vi "2_AdvancedDemo_MHHisto.vi"() -> ()   [LabVIEW 2017]
uses:
  Types/MH_InputChannel.ctl
  Types/MH_UIThread_Cmds.ctl
  Types/MH_UIThread_Data.ctl
  _lib/PQ/MultiHarp/MH_InitInfo.ctl
  Types/MH_SetInpChanData.ctl
  Types/MH_SetInpChanCmds.ctl
  _lib/PQ/MultiHarp/MH_RefSource.ctl
  _lib/PQ/MultiHarp/MH_MeasMode.ctl
  <vilib>/Utility/error.llb/DialogType.ctl
  <vilib>/Utility/error.llb/Error Cluster From Error Code.vi
  _lib/PQ/MultiHarp/MH_LibVersion_global.vi
  _lib/PQ/MultiHarp/mhlib_x86_x64_UIThread.llb/MH_DllPath_global.vi
  <vilib>/ErrorRing/Error Ring.xnode
panel:
  in  "Settings":bool=TRUE
  in  "Run continuously":bool=TRUE caption="Conti."
  in  "Start":bool
  in  "Scale":bool
  out "CountRates":i32[](graph)
  in  "AllChannels":T1={"Enable"=TRUE, "Offset"=0, "Level"=-100, "Edge"=0, "DeadTime"=1000, "UseDeadTime"=FALSE, "SetEnableAllChan"=TRUE, "SetEdgeAllChan"=TRUE, "SetLevelAllChan"=TRUE, "SetOffsetAllChan"=TRUE, "SetUseDTAllChan"=TRUE, "SetDeadTAllChan"=TRUE} {"DeadTime" min=800 max=160000 step=1; "Edge" items=["falling", "rising"]; "Offset" min=-100000 max=100000 step=10; "Level" min=-1200 max=1200 step=1}
  in  "HistoLength":i32(ring)=6 caption="Num Bins" items=["1024", "2048", "4096", "8192", "16384", "32768", "65536"]
  in  "OvlLevel":u32=4294967295 caption="Ovl.Level" min=1 step=1
  in  "StopOvl.":bool=TRUE
  in  "AcqTime":i32=1000 caption="Acqu.           ms" min=1 max=360000 step=1
  in  "Binning":i32(ring) caption="Resol.            ps" items=["10", "20", "40", "80", "160", "320", "640", "1280", "2560", "5120", "10240", "20480", "40960", "81920", "163840", "327680", "655360", "1310720", "2621440", "5242880", "10485760", "20971520", "41943040"]
  in  "HistoOffset":i32 caption="Offset            ns" min=0 max=100000000 step=1
  out "HistoGraph":T2(graph)={0.0, "Resolution"=0.08, "Histogram"=[]}
  in  "SyncDeadTime":i32=1000 caption="Dead T.   ps" min=800 max=160000 step=1
  in  "UseDeadTime":bool caption="Use DT."
  in  "SyncEdge":i32(ring) caption="Edge" items=["falling", "rising"]
  in  "SyncDivider":i32(ring) caption="Divider" items=["1", "2", "4", "8", "16"]
  in  "SyncOffset":i32 caption="Offset      ps" min=-100000 max=100000 step=10
  in  "SyncLevel":i32=-100 caption="Level      mV" min=-1200 max=1200 step=1
  in  "Channels":T3[](array[typedef])=[{"Name"="Inp.Chan 1", "Enable"=TRUE, "Edge"=0, "Level"=-100, "Offset"=0, "UseDeadTime"=FALSE, "DeadTime"=1000}, {"Name"="Inp.Chan 2", "Enable"=TRUE, "Edge"=0, "Level"=-100, "Offset"=0, "UseDeadTime"=FALSE, "DeadTime"=1000}, {"Name"="Inp.Chan 3", "Enable"=TRUE, "Edge"=0, "Level"=-100, "Offset"=0, "UseDeadTime"=FALSE, "DeadTime"=1000}, {"Name"="Inp.Chan 4", "Enable"=TRUE, "Edge"=0, "Level"=-100, "Offset"=0, "UseDeadTime"=FALSE, "DeadTime"=1000}, {"Name"="Inp.Chan 5", "Enable"=TRUE, "Edge"=0, "Level"=-100, "Offset"=0, "UseDeadTime"=FALSE, "DeadTime"=1000}, {"Name"="Inp.Chan 6", "Enable"=TRUE, "Edge"=0, "Level"=-100, "Offset"=0, "UseDeadTime"=FALSE, "DeadTime"=1000}, {"Name"="Inp.Chan 7", "Enable"=TRUE, "Edge"=0, "Level"=-100, "Offset"=0, "UseDeadTime"=FALSE, "DeadTime"=1000}, {"Name"="Inp.Chan 8", "Enable"=TRUE, "Edge"=0, "Level"=-100, "Offset"=0, "UseDeadTime"=FALSE, "DeadTime"=1000}, {"Name"="Inp.Chan 9", "Enable"=TRUE, "Edge"=0, "Level"=-100, "Offset"=0, "UseDeadTime"=FALSE, "DeadTime"=1000}, {"Name"="Inp.Chan 10", "Enable"=TRUE, "Edge"=0, "Level"=-100, "Offset"=0, "UseDeadTime"=FALSE, "DeadTime"=1000}, {"Name"="Inp.Chan 11", "Enable"=TRUE, "Edge"=0, "Level"=-100, "Offset"=0, "UseDeadTime"=FALSE, "DeadTime"=1000}, {"Name"="Inp.Chan 12", "Enable"=TRUE, "Edge"=0, "Level"=-100, "Offset"=0, "UseDeadTime"=FALSE, "DeadTime"=1000}, {"Name"="Inp.Chan 13", "Enable"=TRUE, "Edge"=0, "Level"=-100, "Offset"=0, "UseDeadTime"=FALSE, "DeadTime"=1000}, {"Name"="Inp.Chan 14", "Enable"=TRUE, "Edge"=0, "Level"=-100, "Offset"=0, "UseDeadTime"=FALSE, "DeadTime"=1000}, {"Name"="Inp.Chan 15", "Enable"=TRUE, "Edge"=0, "Level"=-100, "Offset"=0, "UseDeadTime"=FALSE, "DeadTime"=1000}, {"Name"="Inp.Chan 16", "Enable"=TRUE, "Edge"=0, "Level"=-100, "Offset"=0, "UseDeadTime"=FALSE, "DeadTime"=1000}] {"DeadTime" min=800 max=160000 step=1; "Edge" items=["falling", "rising"]; "Offset" min=-100000 max=100000 step=10; "Level" min=-1200 max=1200 step=1}
  out "SyncRate":string="Sync Rate: 4999950 cps\n"
  out "OverFlow":bool caption="Overflow:"
  out "Status":string="Readout Rate: 8.6 Hz\t\tTotal Counts:\t\tCh. 1: 0 cnts.\t\tCh. 2: 1962112 cnts.\t\tCh. 3: 0 cnts.\t\tCh. 4: 1962112 cnts.\t\tCh. 5: 0 cnts.\t\tCh. 6: 1962112 cnts.\t\tCh. 7: 0 cnts.\t\tCh. 8: 1962112 cnts.\t\tCh. 9: 1962113 cnts.\t\tCh.10: 0 cnts.\t\tCh.11: 1962113 cnts.\t\tCh.12: 0 cnts.\t\tCh.13: 1962113 cnts.\t\tCh.14: 0 cnts.\t\tCh.15: 1962113 cnts.\t\tCh.16: 1962113 cnts.\t\t"
  # "Acquisition"
  # "All Channels"
  # "Sync"
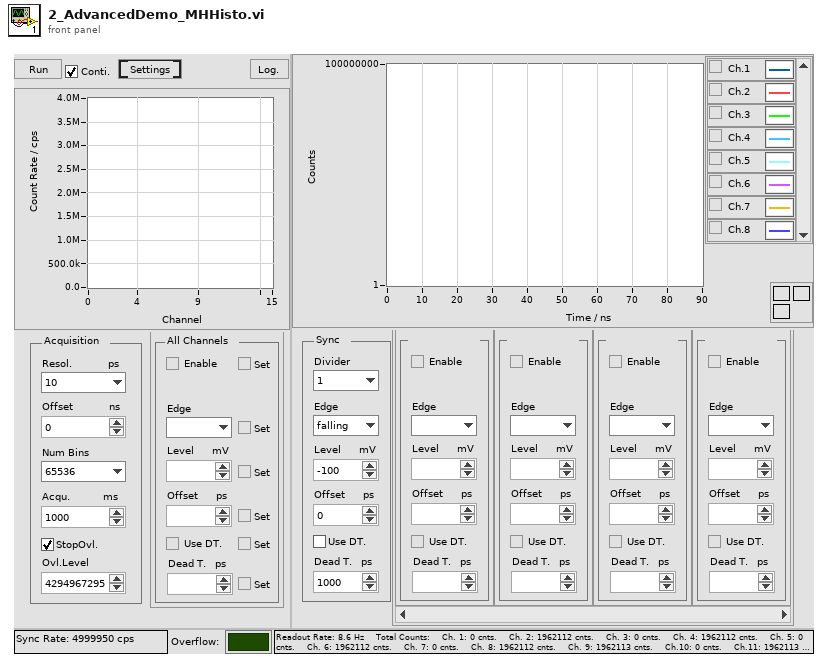
[diagram p1: front panel]
types:
  T1 = cluster{"Enable":bool, "Offset":i32, "Level":i32, "Edge":i32, "DeadTime":i32, "UseDeadTime":bool, "SetEnableAllChan":bool, "SetEdgeAllChan":bool, "SetLevelAllChan":bool, "SetOffsetAllChan":bool, "SetUseDTAllChan":bool, "SetDeadTAllChan":bool}
  T2 = cluster{dbl, "Resolution":dbl, "Histogram":u32[][]}
  T3 = typedef "MH_InputChannel.ctl" = cluster{"Name":string, "Enable":bool, "Edge":i32, "Level":i32, "Offset":i32, "UseDeadTime":bool, "DeadTime":i32}
  T4 = typedef "MH_UIThread_Data.ctl" = cluster{"Init Info":T5, "DevIdx":i32, "SyncDivider":i32, "SyncOffset":i32, "SyncLevel":i32, "Channels":T3[], "CurrentChannels":i32[], "AcqTime":i32, "Binning":i32, "HistoOffset":i32, "HistoLen":i32, "StopOvl.":bool, "OvlLevel":u32, "SyncEdge":i32, "StartMeas":bool, "HistoLength":i32, "Resolution":dbl, "Run cont.":bool, "Status":string, "SyncRate":i32, "BitShift":i32, "HistoAcqTime":dbl, "SyncRateStart":i32, "UseDeadTime":bool, "SyncDeadTime":i32, "SetInpChan":T6[]}
  T5 = typedef "MH_InitInfo.ctl" = cluster{"Library Version":string, "Serial No.":string, "Model":string, "Partnum":string, "Version":string, "features":i32, "nchannels":i32, "Base Resolution":dbl, "Bin Steps":i32}
  T6 = typedef "MH_SetInpChanData.ctl" = cluster{"Channel":i32, "Cmds":T7[], "Changed":cluster{"Name":bool, "Enable":bool, "Edge":bool, "Level":bool, "Offset":bool, "UseDeadTime":bool, "DeadTime":bool}}
  T7 = typedef "MH_SetInpChanCmds.ctl" = enum16{"SetInpChanEnable", "SetInpChanOffset", "SetInpChanDeadTime", "SetInpChanTrg"}
  T8 = typedef "MH_UIThread_Cmds.ctl" = enum16{"Idle", "Init", "SetInpChan", "SetSyncDivider", "SetSyncTrg", "SetSyncOffset", "SetSyncDeadTime", "SetBinning", "SetHistoOffset", "SetHistoLen", "SetStopOvl", "SetBitShift", "SetHistoAcqTime", "GetRates", "GetAllRates", "StartMeas", "StopMeas", "AbortMeas", "GetResolution", "GetHistos", "GetAllHistos", "ReadFiFo", "WriteStatus", "Resize", "EnableControls", "DisableControls", "Error", "Exit"}
  T9 = enum8{"Enabled", "Disabled", "Disabled and Grayed Out"}
  T10 = cluster{"[0]":bool, "[1]":bool, "[2]":bool, "[3]":bool, "[4]":bool, "[5]":bool}
  T11 = typedef "MH_MeasMode.ctl" = i32
  T12 = typedef "MH_RefSource.ctl" = enum16{"INTERNAL", "EXTERNAL_10MHZ", "WR_MASTER_GENERIC", "WR_SLAVE_GENERIC", "WR_GRANDM_GENERIC", "EXTN_GPS_PPS", "EXTN_GPS_PPS_UART", "WR_MASTER_MHARP", "WR_SLAVE_MHARP", "WR_GRANDM_MHARP"}
  T13 = cluster{dbl, "Resolution":dbl, "Histograms":u32[][]}
  T14 = typedef "DialogType.ctl" = u16
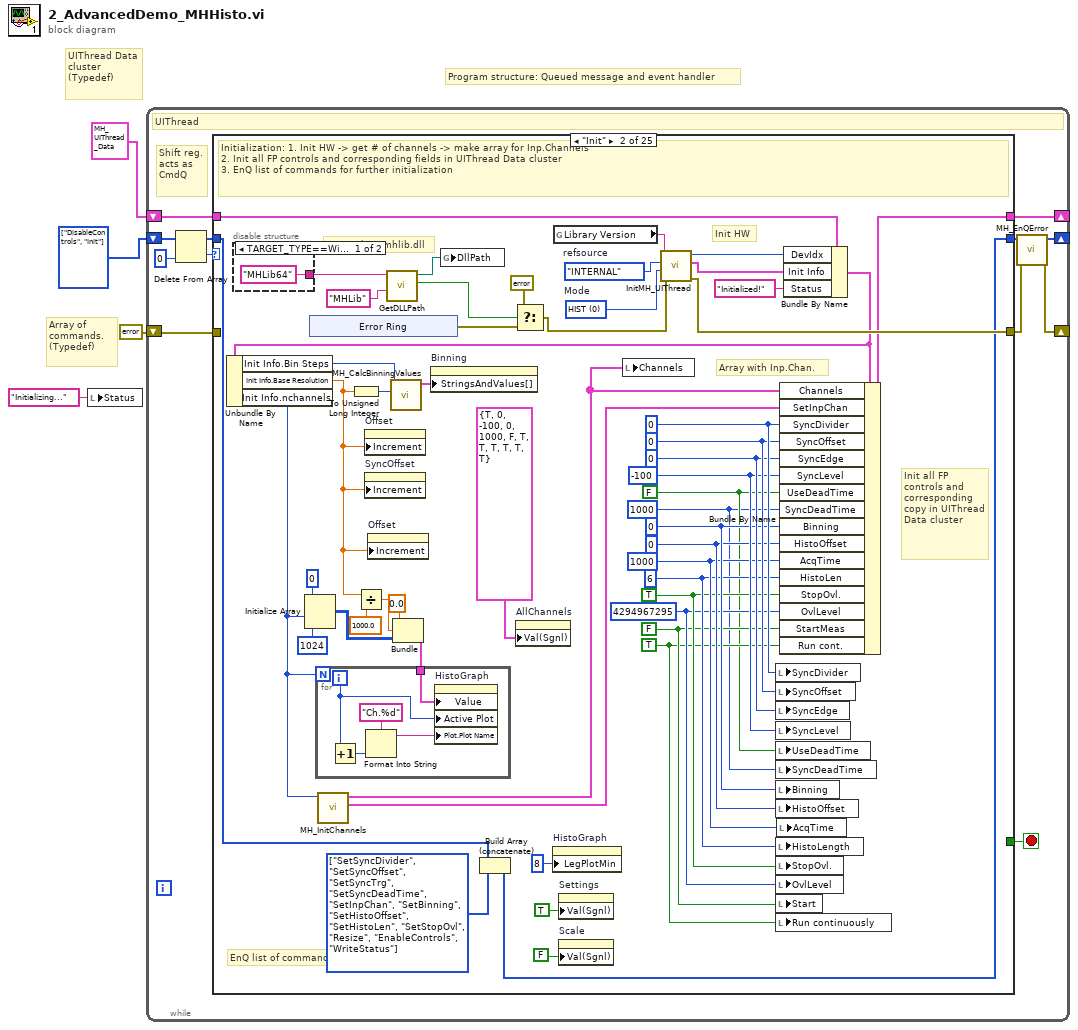
[diagram p0: block diagram]
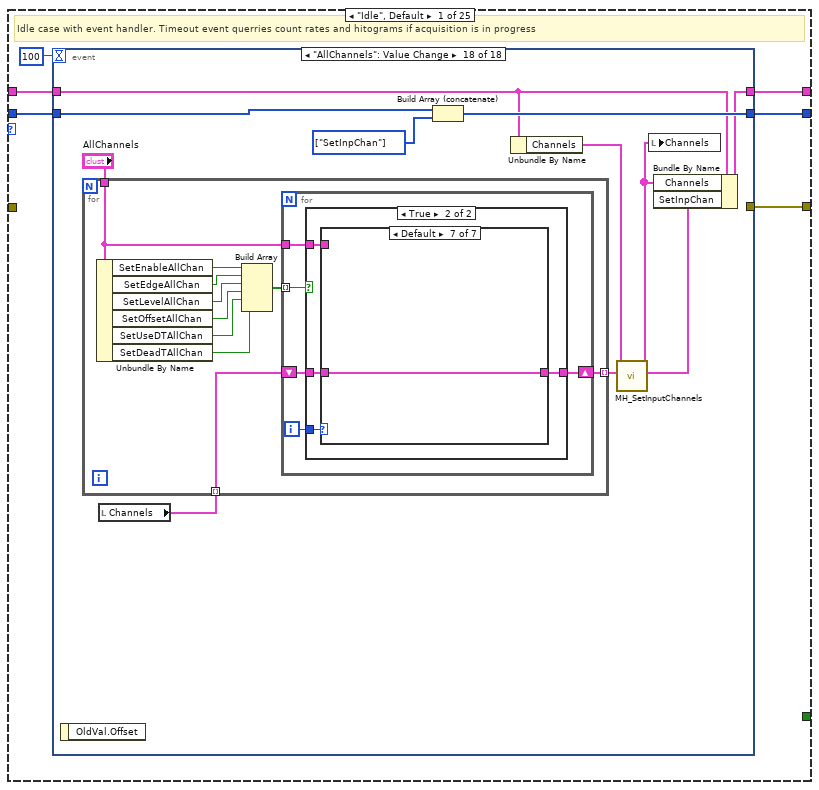
[diagram p2: hidden frame]
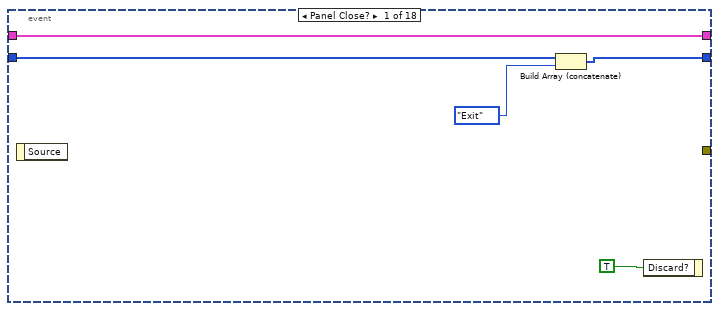
[diagram p3: hidden frame]
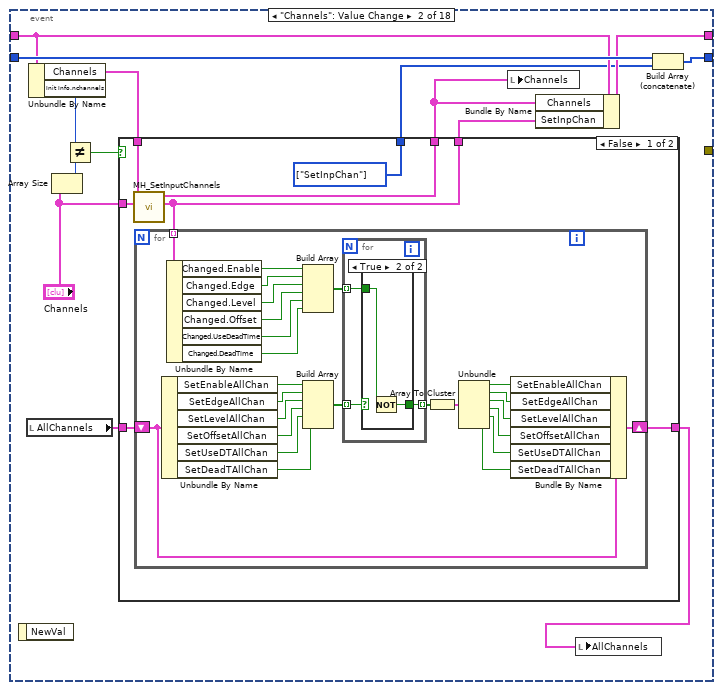
[diagram p4: hidden frame]
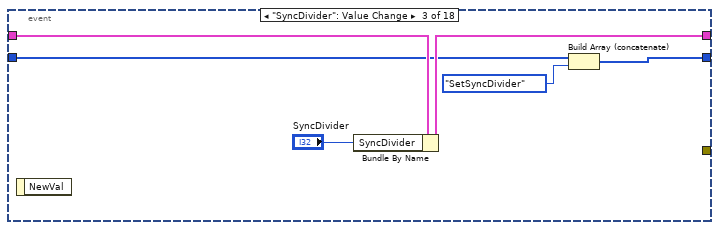
[diagram p7: hidden frame]
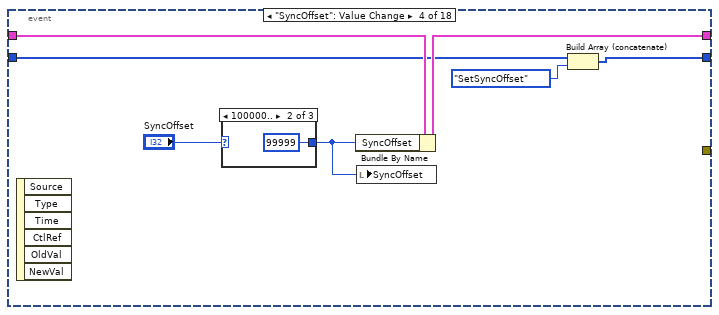
[diagram p8: hidden frame]
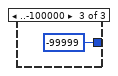
[diagram p10: hidden frame]
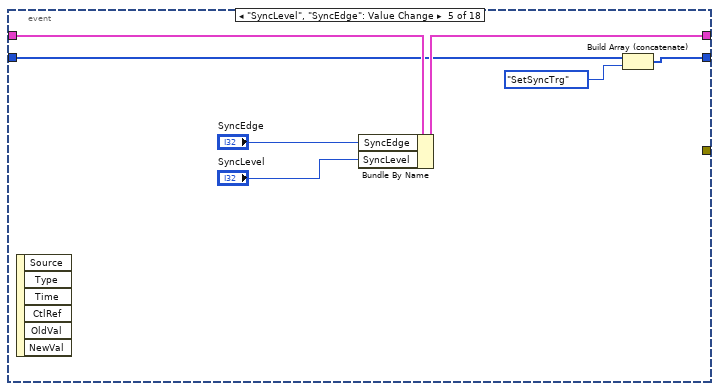
[diagram p11: hidden frame]
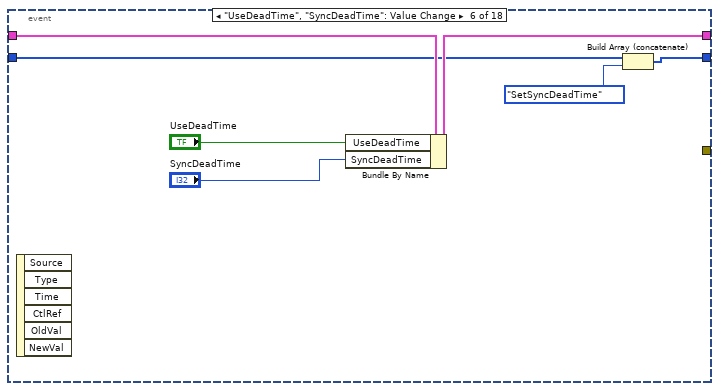
[diagram p12: hidden frame]
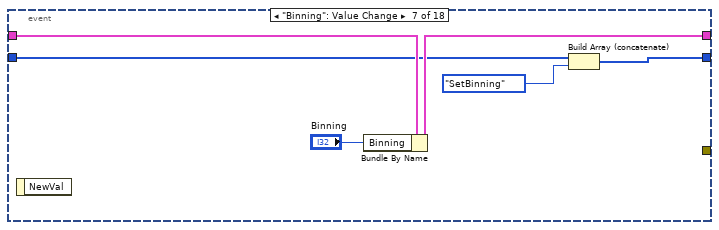
[diagram p13: hidden frame]
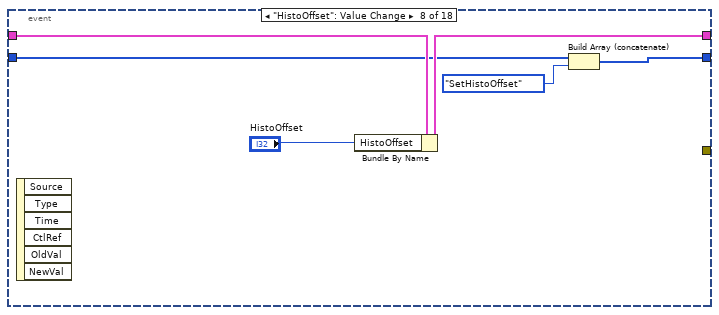
[diagram p14: hidden frame]
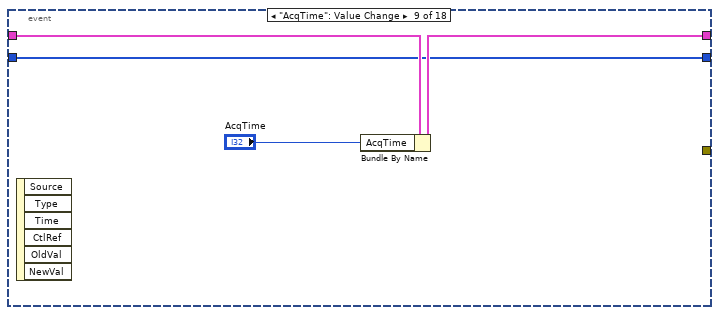
[diagram p15: hidden frame]
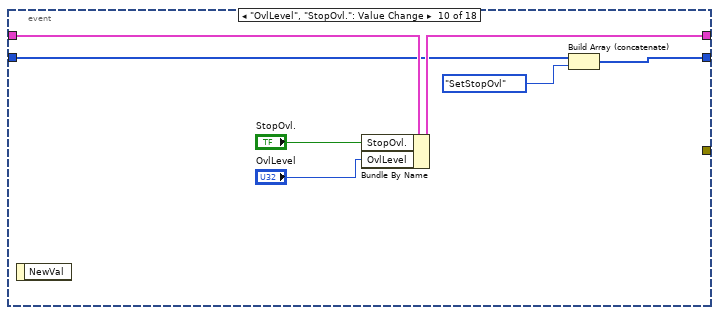
[diagram p16: hidden frame]
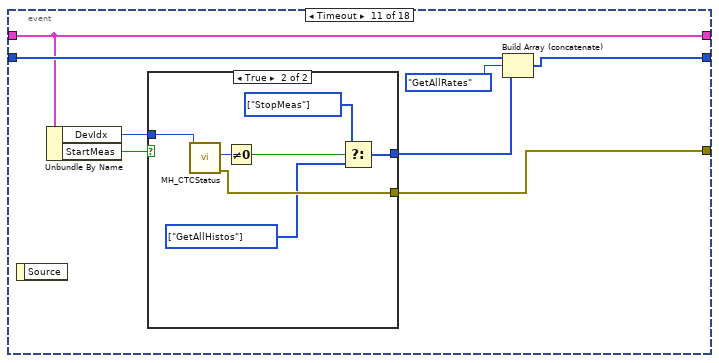
[diagram p17: hidden frame]
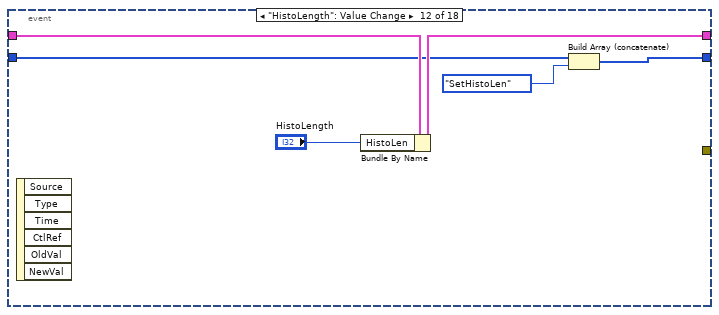
[diagram p19: hidden frame]
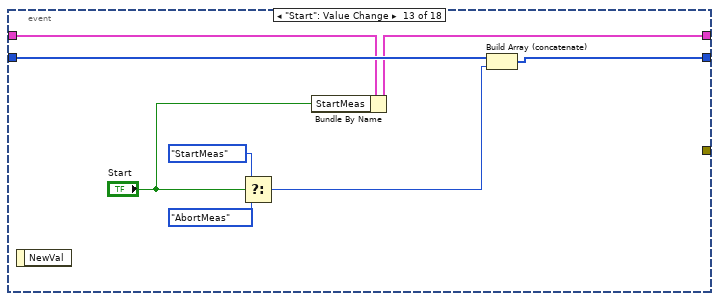
[diagram p20: hidden frame]
diagram:
  w3 = T8[] [enum."DisableControls", enum."Init"] items=["Idle", "Init", "SetInpChan", "SetSyncDivider", "SetSyncTrg", "SetSyncOffset", "SetSyncDeadTime", "SetBinning", "SetHistoOffset", "SetHistoLen", "SetStopOvl", "SetBitShift", "SetHistoAcqTime", "GetRates", "GetAllRates", "StartMeas", "StopMeas", "AbortMeas", "GetResolution", "GetHistos", "GetAllHistos", "ReadFiFo", "WriteStatus", "Resize", "EnableControls", "DisableControls", "Error", "Exit"]
  # "Array of commands.\n(Typedef)"
  # "Program structure: Queued message and event handler"
  # "UIThread Data cluster\n(Typedef)"
  n1 = local write "Status"("Initializing..." ("Status")) -> ()
  n2 = while {
    shift-right: [w5] -> _
    shift-left: w3 -> [w12]
    shift-right: [w15] -> _
    shift-left: T4 {"Init Info"={"Library Version"="", "Serial No."="", "Model"="", "Partnum"="", "Version"="", "features"=0, "nchannels"=0, "Base Resolution"=0.0, "Bin Steps"=0}, "DevIdx"=0, "SyncDivider"=1, "SyncOffset"=0, "SyncLevel"=50, "Channels"=[], "CurrentChannels"=[], "AcqTime"=1, "Binning"=1, "HistoOffset"=1, "HistoLen"=1024, "StopOvl."=FALSE, "OvlLevel"=1024, "SyncEdge"=10, "StartMeas"=FALSE, "HistoLength"=0, "Resolution"=0.0, "Run cont."=FALSE, "Status"="", "SyncRate"=0, "BitShift"=0, "HistoAcqTime"=0.0, "SyncRateStart"=0, "UseDeadTime"=FALSE, "SyncDeadTime"=800, "SetInpChan"=[]} -> [w14]
    shift-right: [w7] -> _
    shift-left: errorcluster {"status"=FALSE, "code"=0, "source"=""} ("error IO") -> [w13]
    stop <- w16 stop-if-true
    # "Shift reg.\nacts as\nCmdQ"
    # "UIThread"
    n3 = Delete From Array(array=w12, index=0) -> (deleted portion=w10:T8, array with subset deleted=w9:T8[])  [unwired: 1 in]
    n4 = case shown="\"Init\"" w10 {
      tunnel: [w22 w301 w325 w387 w396 w408 w414 w421 w429 w437 w442 w453 w464 w479 w487 w501 w515 w540 w572 w596 w609 w616 w628 w634 w638] -> w6
      tunnel: [_ _ _ _ _ _ _ _ _ _ _ _ _ _ _ _ _ _ _ _ _ _ _ _ TRUE] -> w16
      tunnel: [w21 w281 w326 w389 w397 w409 w418 w425 w430 w432 w443 w452 w463 w485 w490 w504 w511 w539 w571 w595 w597 w615 w627 w635 w641] -> w15
      tunnel: w14 -> [w20 w286 w326 w389 w397 w409 w418 w425 w430 w433 w443 w452 w463 w485 w491 w505 w512 w539 w571 w595 w597 w615 w627 w635 w641]
      tunnel: [w17 w304 w323 w385 w395 w407 w417 w424 w428 w436 w441 w446 w462 w484 w493 w507 w513 w537 w567 _ _ _ _ _ w639] -> w8
      tunnel: w13 -> [_ _ _ _ _ _ _ _ _ _ _ _ _ _ _ _ _ _ _ _ _ _ _ w636 _]
      tunnel: w9 -> [w19 w303 w325 w387 w396 w408 w414 w420 w429 w437 w442 w453 w464 w480 w488 w502 w515 w540 w572 w596 w609 w616 w628 _ w638]
      frame "Idle", Default {
        # "Idle case with event handler. Timeout event querries count rates and hitograms if acquisition is in progress"
        n5 = event shown="[17] \"AllChannels\": Value Change" {
          selector: _ -> [_ _ _ _ _ _ _ _ _ _ _ _ _ _ _ _ _ _]
          dyn-events: _ -> [_ _ _ _ _ _ _ _ _ _ _ _ _ _ _ _ _ _]
          timeout: 100 -> [_ _ _ _ _ _ _ _ _ _ _ _ _ _ _ _ _ _]
          tunnel: [w23 w40 w82 w90 w99 w107 w113 w119 w124 w130 w140 w151 w159 w167 w173 w181 w191 w204] -> w22
          tunnel: [w26 w33 w86 w93 w103 w110 w116 w122 w126 w133 w139 w154 w157 w165 w172 w180 w194 w198] -> w21
          tunnel: w20 -> [w26 w35 w87 w94 w104 w111 w117 w123 w127 w134 w139 w155 w158 w166 w172 w180 w194 w199]
          tunnel: w19 -> [w25 w41 w84 w92 w101 w109 w115 w121 w124 w132 w142 w153 w161 w167 w173 w181 w192 w205]
          tunnel: [_ _ _ _ _ _ _ _ _ _ w135 _ _ _ _ _ _ _] -> w17
          event Panel Close? {
            n6 = event-data() -> ()  [unwired: 1 in, 1 out]
            n7 = Build Array (concatenate)(w25, MH_UIThread_Cmds."Exit") -> (w23:T8[])
            n8 = event-data("Discard?"=TRUE) -> ()  [unwired: 1 in, 1 out]
          }
          event "Channels": Value Change {
            n9 = event-data() -> ()  [unwired: 1 in, 1 out]
            n10 = local read "AllChannels"() -> (w29:T1)
            n11 = Unbundle By Name(w35) -> ("Channels"=w36:T3[], "Init Info.nchannels"=w39:i32)
            n12 = Array Size(array="Channels") -> (size(s)=w38:i32)
            n13 = Not Equal?(x=w39, y=w38) -> (x != y?=w37:bool)
            n14 = case shown="False" w37 {
              tunnel: "Channels" -> [w47 _]
              tunnel: [w46 w81] -> w34
              tunnel: w36 -> [w48 w81]
              tunnel: [w44 _] -> w32
              tunnel: [w45 _] -> w30
              tunnel: w29 -> [w43 w80]
              tunnel: [w42 w80] -> w28
              frame False {
                w45 = T8[] [enum."SetInpChan"] items=["Idle", "Init", "SetInpChan", "SetSyncDivider", "SetSyncTrg", "SetSyncOffset", "SetSyncDeadTime", "SetBinning", "SetHistoOffset", "SetHistoLen", "SetStopOvl", "SetBitShift", "SetHistoAcqTime", "GetRates", "GetAllRates", "StartMeas", "StopMeas", "AbortMeas", "GetResolution", "GetHistos", "GetAllHistos", "ReadFiFo", "WriteStatus", "Resize", "EnableControls", "DisableControls", "Error", "Exit"] ("array")
                n15 = call "MH_SetInputChannels.vi"("Channels new"=w47, "Channels old"=w48) -> ("SetInpChan"=w44:T6[], "Channels"=w46:T3[])  [unwired: 8 in]
                n16 = for {
                  tunnel: w44 -> [w73] mode=indexing
                  shift-right: [w55] -> w42
                  shift-left: w43 -> [w57]
                  n17 = Unbundle By Name(w57) -> ("SetEnableAllChan"=w66:bool, "SetEdgeAllChan"=w65:bool, "SetLevelAllChan"=w64:bool, "SetOffsetAllChan"=w63:bool, "SetUseDTAllChan"=w62:bool, "SetDeadTAllChan"=w61:bool)
                  n18 = Unbundle By Name(w73) -> ("Changed.Enable"=w72:bool, "Changed.Edge"=w71:bool, "Changed.Level"=w70:bool, "Changed.Offset"=w69:bool, "Changed.UseDeadTime"=w68:bool, "Changed.DeadTime"=w67:bool)
                  n19 = Build Array(w72, w71, w70, w69, w68, w67) -> (w59:bool[])
                  n20 = Build Array(w66, w65, w64, w63, w62, w61) -> (w60:bool[])
                  n21 = for {
                    tunnel: w60 -> [w76] mode=indexing
                    tunnel: w59 -> [w74] mode=indexing
                    tunnel: [w75] -> w58 mode=indexing
                    n22 = case shown="True" w76 {
                      selector: w76 -> [w77 _]
                      tunnel: [w77 w78] -> w75
                      tunnel: w74 -> [_ w79]
                      frame False {
                      }
                      frame True {
                        n23 = Not(x=w79) -> (.not. x?=w78:bool)
                      }
                    }
                  }
                  n24 = Array To Cluster(array=w58) -> (cluster=w56:T10)
                  n25 = Unbundle(w56) -> ("[0]"=w54:bool, "[1]"=w53:bool, "[2]"=w52:bool, "[3]"=w51:bool, "[4]"=w50:bool, "[5]"=w49:bool)
                  n26 = Bundle By Name(cluster=w57, "SetEnableAllChan"=w54, "SetEdgeAllChan"=w53, "SetLevelAllChan"=w52, "SetOffsetAllChan"=w51, "SetUseDTAllChan"=w50, "SetDeadTAllChan"=w49) -> (w55:T1)
                }
              }
              frame True {
              }
            }
            n27 = local write "Channels"(w34) -> ()
            n28 = Bundle By Name(cluster=w35, "Channels"=w34, "SetInpChan"=w32) -> (w33:T4)
            n29 = local write "AllChannels"(w28) -> ()
            n30 = Build Array (concatenate)(w41, w30) -> (w40:T8[])
          }
          event "SyncDivider": Value Change {
            n31 = event-data() -> ()  [unwired: 1 in, 1 out]
            n32 = Bundle By Name(cluster=w87, "SyncDivider"="SyncDivider") -> (w86:T4)
            n33 = Build Array (concatenate)(w84, MH_UIThread_Cmds."SetSyncDivider") -> (w82:T8[])
          }
          event "SyncOffset": Value Change {
            n34 = event-data() -> ()  [unwired: 1 in, 6 out]
            n35 = case shown="100000.." "SyncOffset" {
              selector: "SyncOffset" -> [w95 _ _]
              tunnel: [w95 99999 ("SyncOffset") -99999 ("SyncOffset")] -> w88
              frame Default {
              }
              frame 100000.. {
              }
              frame ..-100000 {
              }
            }
            n36 = Bundle By Name(cluster=w94, "SyncOffset"=w88) -> (w93:T4)
            n37 = local write "SyncOffset"(w88) -> ()
            n38 = Build Array (concatenate)(w92, MH_UIThread_Cmds."SetSyncOffset") -> (w90:T8[])
          }
          event "SyncLevel", "SyncEdge": Value Change {
            n39 = event-data() -> ()  [unwired: 1 in, 6 out]
            n40 = Bundle By Name(cluster=w104, "SyncEdge"="SyncEdge", "SyncLevel"="SyncLevel") -> (w103:T4)
            n41 = Build Array (concatenate)(w101, MH_UIThread_Cmds."SetSyncTrg") -> (w99:T8[])
          }
          event "UseDeadTime", "SyncDeadTime": Value Change {
            n42 = event-data() -> ()  [unwired: 1 in, 6 out]
            n43 = Bundle By Name(cluster=w111, "UseDeadTime"="UseDeadTime", "SyncDeadTime"="SyncDeadTime") -> (w110:T4)
            n44 = Build Array (concatenate)(w109, MH_UIThread_Cmds."SetSyncDeadTime") -> (w107:T8[])
          }
          event "Binning": Value Change {
            n45 = event-data() -> ()  [unwired: 1 in, 1 out]
            n46 = Bundle By Name(cluster=w117, "Binning"="Binning") -> (w116:T4)
            n47 = Build Array (concatenate)(w115, MH_UIThread_Cmds."SetBinning") -> (w113:T8[])
          }
          event "HistoOffset": Value Change {
            n48 = event-data() -> ()  [unwired: 1 in, 6 out]
            n49 = Bundle By Name(cluster=w123, "HistoOffset"="HistoOffset") -> (w122:T4)
            n50 = Build Array (concatenate)(w121, MH_UIThread_Cmds."SetHistoOffset") -> (w119:T8[])
          }
          event "AcqTime": Value Change {
            n51 = event-data() -> ()  [unwired: 1 in, 6 out]
            n52 = Bundle By Name(cluster=w127, "AcqTime"="AcqTime") -> (w126:T4)
          }
          event "OvlLevel", "StopOvl.": Value Change {
            n53 = event-data() -> ()  [unwired: 1 in, 1 out]
            n54 = Bundle By Name(cluster=w134, "StopOvl."="StopOvl.", "OvlLevel"="OvlLevel") -> (w133:T4)
            n55 = Build Array (concatenate)(w132, MH_UIThread_Cmds."SetStopOvl") -> (w130:T8[])
          }
          event Timeout {
            n56 = event-data() -> ()  [unwired: 1 in, 1 out]
            n57 = Unbundle By Name(w139) -> ("DevIdx"=w137:i32, "StartMeas"=w138:bool)
            n58 = case shown="True" w138 {
              tunnel: w137 -> [_ w149]
              tunnel: [_ w147] -> w136
              tunnel: [_ w145] -> w135
              frame False {
              }
              frame True {
                w143 = T8[] [enum."GetAllHistos"] items=["Idle", "Init", "SetInpChan", "SetSyncDivider", "SetSyncTrg", "SetSyncOffset", "SetSyncDeadTime", "SetBinning", "SetHistoOffset", "SetHistoLen", "SetStopOvl", "SetBitShift", "SetHistoAcqTime", "GetRates", "GetAllRates", "StartMeas", "StopMeas", "AbortMeas", "GetResolution", "GetHistos", "GetAllHistos", "ReadFiFo", "WriteStatus", "Resize", "EnableControls", "DisableControls", "Error", "Exit"]
                w146 = T8[] [enum."StopMeas"] items=["Idle", "Init", "SetInpChan", "SetSyncDivider", "SetSyncTrg", "SetSyncOffset", "SetSyncDeadTime", "SetBinning", "SetHistoOffset", "SetHistoLen", "SetStopOvl", "SetBitShift", "SetHistoAcqTime", "GetRates", "GetAllRates", "StartMeas", "StopMeas", "AbortMeas", "GetResolution", "GetHistos", "GetAllHistos", "ReadFiFo", "WriteStatus", "Resize", "EnableControls", "DisableControls", "Error", "Exit"]
                n59 = call "MH_CTCStatus.vi"("devidx"=w149) -> ("error out"=w145:errorcluster, "ctcstatus"=w148:i32)  [unwired: 8 in, 1 out]
                n60 = Not Equal To 0?(x=w148) -> (x != 0?=w144:bool)
                n61 = Select(t=w146, s=w144, f=w143) -> (s? t:f=w147:T8[])
              }
            }
            n62 = Build Array (concatenate)(w142, MH_UIThread_Cmds."GetAllRates", w136) -> (w140:T8[])
          }
          event "HistoLength": Value Change {
            n63 = event-data() -> ()  [unwired: 1 in, 6 out]
            n64 = Bundle By Name(cluster=w155, "HistoLen"="HistoLength") -> (w154:T4)
            n65 = Build Array (concatenate)(w153, MH_UIThread_Cmds."SetHistoLen") -> (w151:T8[])
          }
          event "Start": Value Change {
            n66 = event-data() -> ()  [unwired: 1 in, 1 out]
            n67 = Select(t=MH_UIThread_Cmds."StartMeas", s="Start", f=MH_UIThread_Cmds."AbortMeas") -> (s? t:f=w160:T8)
            n68 = Bundle By Name(cluster=w158, "StartMeas"="Start") -> (w157:T4)
            n69 = Build Array (concatenate)(w161, w160) -> (w159:T8[])
          }
          event "Run continuously": Value Change {
            n70 = event-data() -> ()  [unwired: 1 in, 1 out]
            n71 = Bundle By Name(cluster=w166, "Run cont."="Run continuously") -> (w165:T4)
          }
          event "Scale": Value Change {
            n72 = event-data() -> ()  [unwired: 1 in, 1 out]
            n73 = Select(t=u8 0 ("Y Scale.Mapping Mode"), s="Scale", f=u8 1 ("Y Scale.Mapping Mode")) -> (s? t:f=w168:u8)
            n74 = property on="HistoGraph" class="WFGraph (strict)"("YScale.Mapping Mode"=w168) -> ()  [unwired: 2 in, 2 out]
          }
          event "Settings": Value Change {
            n75 = event-data() -> ()  [unwired: 1 in, 1 out]
            n76 = property on="Splitter" class="Splitter"() -> ("Position"=w179:i32)  [unwired: 2 in, 2 out]
            n77 = Select(t=300 ("PosT"), s="Settings", f=0 ("PosF")) -> (s? t:f=w176:i32)
            n78 = Subtract(x=w179, y=w176) -> (x-y=w175:i32)
            n79 = while {
              shift-right: [w190] -> _
              shift-left: w175 -> [w183]
              i -> [w189]
              stop <- w186 stop-if-true
              n80 = property on="Splitter 4" class="Splitter"("Position"=w183) -> (error out=w182:errorcluster)  [unwired: 2 in, 1 out]
              n81 = Greater Or Equal?(x=w189, y=10) -> (x >= y?=w187:bool)
              n82 = Decrement(x=w183) -> (x-1=w190:i32)
              n83 = Unbundle(w182) -> ("status"=w185:bool)  [unwired: 2 out]
              n84 = Not(x=w185) -> (.not. x?=w184:bool)
              n85 = Or(x=w184, y=w187) -> (x .or. y?=w186:bool)
            }
          }
          event Panel Resize {
            n86 = event-data() -> ()  [unwired: 1 in, 1 out]
            n87 = Build Array (concatenate)(w192, MH_UIThread_Cmds."Resize") -> (w191:T8[])
          }
          event "AllChannels": Value Change {
            w196 = T8[] [enum."SetInpChan"] items=["Idle", "Init", "SetInpChan", "SetSyncDivider", "SetSyncTrg", "SetSyncOffset", "SetSyncDeadTime", "SetBinning", "SetHistoOffset", "SetHistoLen", "SetStopOvl", "SetBitShift", "SetHistoAcqTime", "GetRates", "GetAllRates", "StartMeas", "StopMeas", "AbortMeas", "GetResolution", "GetHistos", "GetAllHistos", "ReadFiFo", "WriteStatus", "Resize", "EnableControls", "DisableControls", "Error", "Exit"] ("array")
            n88 = event-data() -> ()  [unwired: 1 in, 1 out]
            n89 = local read "Channels"() -> (w203:T3[])
            n90 = for {
              tunnel: w203 -> [w208] mode=indexing
              tunnel: "AllChannels" -> [w207]
              tunnel: [w206] -> w201 mode=indexing
              n91 = Unbundle By Name(w207) -> ("SetEnableAllChan"=w209:bool, "SetEdgeAllChan"=w210:bool, "SetLevelAllChan"=w211:bool, "SetOffsetAllChan"=w212:bool, "SetUseDTAllChan"=w213:bool, "SetDeadTAllChan"=w214:bool)
              n92 = Build Array(w209, w210, w211, w212, w213, w214) -> (w215:bool[])
              n93 = for {
                tunnel: w215 -> [w220] mode=indexing
                shift-right: [w217] -> w206
                shift-left: w208 -> [w218]
                tunnel: w207 -> [w216]
                i -> [w219]
                n94 = case shown="True" w220 {
                  tunnel: w219 -> [_ w225]
                  tunnel: w216 -> [_ w224]
                  tunnel: w218 -> [w221 w223]
                  tunnel: [w221 w222] -> w217
                  frame False {
                  }
                  frame True {
                    n95 = case shown="Default" w225 {
                      tunnel: w224 -> [w229 w233 w237 w242 w249 w253 _]
                      tunnel: w223 -> [w228 w232 w236 w241 w248 w252 w254]
                      tunnel: [w226 w230 w234 w240 w246 w250 w254] -> w222
                      frame 0 {
                        n96 = Unbundle By Name(w229) -> ("Enable"=w227:bool)
                        n97 = Bundle By Name(cluster=w228, "Enable"=w227) -> (w226:T3)
                      }
                      frame 1 {
                        n98 = Unbundle By Name(w233) -> ("Edge"=w231:i32)
                        n99 = Bundle By Name(cluster=w232, "Edge"=w231) -> (w230:T3)
                      }
                      frame 2 {
                        n100 = Unbundle By Name(w237) -> ("Level"=w235:i32)
                        n101 = Bundle By Name(cluster=w236, "Level"=w235) -> (w234:T3)
                      }
                      frame 3 {
                        n102 = Unbundle By Name(w242) -> ("Offset"=w239:i32)
                        n103 = case shown="100000.." w239 {
                          selector: w239 -> [w243 _ _]
                          tunnel: [w243 99999 ("SyncOffset") -99999 ("SyncOffset")] -> w238
                          frame Default {
                          }
                          frame 100000.. {
                          }
                          frame ..-100000 {
                          }
                        }
                        n104 = Bundle By Name(cluster=w241, "Offset"=w238) -> (w240:T3)
                      }
                      frame 4 {
                        n105 = Unbundle By Name(w249) -> ("UseDeadTime"=w247:bool)
                        n106 = Bundle By Name(cluster=w248, "UseDeadTime"=w247) -> (w246:T3)
                      }
                      frame 5 {
                        n107 = Unbundle By Name(w253) -> ("DeadTime"=w251:i32)
                        n108 = Bundle By Name(cluster=w252, "DeadTime"=w251) -> (w250:T3)
                      }
                      frame Default {
                      }
                    }
                  }
                }
              }
            }
            n109 = Build Array (concatenate)(w205, w196) -> (w204:T8[])
            n110 = Unbundle By Name(w199) -> ("Channels"=w200:T3[])
            n111 = call "MH_SetInputChannels.vi"("Channels new"=w201, "Channels old"=w200) -> ("SetInpChan"=w197:T6[], "Channels"=w195:T3[])  [unwired: 8 in]
            n112 = local write "Channels"(w195) -> ()
            n113 = Bundle By Name(cluster=w199, "Channels"=w195, "SetInpChan"=w197) -> (w198:T4)
          }
        }
      }
      frame "Init" {
        w262 = 1000 ("SyncDeadTime")
        w263 = FALSE ("UseDeadTime")
        w265 = T11 0 items=["HIST"=0, "T2"=2, "T3"=3]  # Mode
        w274 = MH_RefSource."INTERNAL"  # refsource
        w288 = TRUE ("Run cont.")
        w290 = FALSE ("StartMeas")
        w291 = u32 4294967295 ("OvlLevel")
        w292 = TRUE ("StopOvl.")
        w293 = 6 ("HistoLen")
        w294 = 1000 ("AcqTime")
        w295 = 0 ("HistoOffset")
        w296 = 0 ("Binning")
        w297 = -100 ("SyncLevel")
        w298 = 0 ("SyncZeroX")
        w299 = 0 ("SyncOffset")
        w300 = 0 ("SyncDivider")
        w302 = T8[] [enum."SetSyncDivider", enum."SetSyncOffset", enum."SetSyncTrg", enum."SetSyncDeadTime", enum."SetInpChan", enum."SetBinning", enum."SetHistoOffset", enum."SetHistoLen", enum."SetStopOvl", enum."Resize", enum."EnableControls", enum."WriteStatus"] items=["Idle", "Init", "SetInpChan", "SetSyncDivider", "SetSyncTrg", "SetSyncOffset", "SetSyncDeadTime", "SetBinning", "SetHistoOffset", "SetHistoLen", "SetStopOvl", "SetBitShift", "SetHistoAcqTime", "GetRates", "GetAllRates", "StartMeas", "StopMeas", "AbortMeas", "GetResolution", "GetHistos", "GetAllHistos", "ReadFiFo", "WriteStatus", "Resize", "EnableControls", "DisableControls", "Error", "Exit"]
        # "Init HW"
        # "Set path to mhlib.dll"
        # "Init all FP controls and corresponding copy in UIThread Data cluster"
        # "EnQ list of commands"
        # "Array with Inp.Chan."
        # "Initialization: 1. Init HW -> get # of channels -> make array for Inp.Channels\n2. Init all FP controls and corresponding fields in UIThread Data cluster\n3. EnQ list of commands for further initialization"
        n114 = disable-structure shown="TARGET_TYPE==Windows, Default" {
          disable-tunnel: ["MHLib64" ("name or relative path") "MHLib" ("name or relative path")] -> w264
          frame condition #0 (active) {
          }
          frame condition #1 {
          }
        }
        n115 = xnode "Error Ring"() -> ("error out"=w275:errorcluster)
        n116 = call "GetDLLPath.vi"("DllName_32bit"="MHLib" ("name or relative path"), "DllName_64bit"=w264) -> ("file exists?"=w277:bool, "DLLPath"=w278:path)  [unwired: 8 in]
        n117 = global write "MH_DllPath_global.vi" "DllPath"(w278) -> ()
        n118 = Build Array (concatenate)(w303, w302) -> (w301:T8[])
        n119 = Select(t=errorcluster {"status"=FALSE, "code"=0, "source"=""} ("error IO"), s=w277, f=w275) -> (s? t:f=w282:errorcluster)
        n120 = property on="AllChannels" class="Clust (strict)"("Val(Sgnl)"=T1 {"Enable"=TRUE, "Offset"=0, "Level"=-100, "Edge"=0, "DeadTime"=1000, "UseDeadTime"=FALSE, "SetEnableAllChan"=TRUE, "SetEdgeAllChan"=TRUE, "SetLevelAllChan"=TRUE, "SetOffsetAllChan"=TRUE, "SetUseDTAllChan"=TRUE, "SetDeadTAllChan"=TRUE} ("AllChannels")) -> ()  [unwired: 2 in, 2 out]
        n121 = property on="HistoGraph" class="WFGraph (strict)"("LegPlotMin"=u32 8 ("Legend:Plot Minimum")) -> ()  [unwired: 2 in, 2 out]
        n122 = global read "MH_LibVersion_global.vi" "Library Version"() -> (w273:string)
        n123 = property on="Settings" class="Bool (strict)"("Val(Sgnl)"=TRUE ("Value (Signaling)")) -> ()  [unwired: 2 in, 2 out]
        n124 = property on="Scale" class="Bool (strict)"("Val(Sgnl)"=FALSE ("Value (Signaling)")) -> ()  [unwired: 2 in, 2 out]
        n125 = call "InitMH_UIThread.vi"("error in (no error)"=w282, "Mode"=w265, "refsource"=w274, "Library Version"=w273) -> ("error out"=w304:errorcluster, "Init Info"=w306:T5, "DevIdx"=w305:i32)  [unwired: 5 in]
        n126 = local write "SyncDivider"(w300) -> ()
        n127 = local write "SyncOffset"(w299) -> ()
        n128 = local write "SyncEdge"(w298) -> ()
        n129 = local write "SyncLevel"(w297) -> ()
        n130 = local write "UseDeadTime"(w263) -> ()
        n131 = local write "SyncDeadTime"(w262) -> ()
        n132 = local write "Binning"(w296) -> ()
        n133 = local write "HistoOffset"(w295) -> ()
        n134 = local write "HistoLength"(w293) -> ()
        n135 = local write "StopOvl."(w292) -> ()
        n136 = local write "OvlLevel"(w291) -> ()
        n137 = local write "Start"(w290) -> ()
        n138 = local write "Run continuously"(w288) -> ()
        n139 = local write "AcqTime"(w294) -> ()
        n140 = Bundle By Name(cluster=w286, "DevIdx"=w305, "Init Info"=w306, "Status"="Initialized!") -> (w285:T4)
        n141 = Unbundle By Name(w285) -> ("Init Info.Bin Steps"=w284:i32, "Init Info.Base Resolution"=w255:dbl, "Init Info.nchannels"=w260:i32)
        n142 = Initialize Array(u32 0, w260, 1024 ("dimension size")) -> (w267:u32[][])
        n143 = call "MH_InitChannels.vi"("nchannels"=w260) -> ("SetInpChan"=w258:T6[], "Channels"=w259:T3[])  [unwired: 9 in]
        n144 = To Unsigned Long Integer(number=w255) -> (unsigned 32bit integer=w256:u32)
        n145 = Divide(x=w255, y=1000.0) -> (x/y=w268:dbl)
        n146 = property on="Offset" class="DigNum (strict)"("Increment"=w255) -> ()  [unwired: 2 in, 2 out]
        n147 = property on="SyncOffset" class="DigNum (strict)"("Increment"=w255) -> ()  [unwired: 2 in, 2 out]
        n148 = property on="Offset" class="DigNum (strict)"("Increment"=w255) -> ()  [unwired: 2 in, 2 out]
        n149 = call "MH_CalcBinningValues.vi"("BaseResolution"=w256, "Bin Steps"=w284) -> ("BinningValues"=w289:cluster{"String":string, "Value":i32}[])  [unwired: 9 in]
        n150 = Bundle(0.0, w268, w267) -> (w261:cluster{dbl, dbl, u32[][]})  [unwired: 1 in]
        n151 = for {
          N: w260 -> [_]
          tunnel: w261 -> [w314]
          i -> [w316]
          n152 = Increment(x=w316) -> (x+1=w315:i32)
          n153 = Format Into String(format string="Ch.%d", w315) -> (resulting string=w317:string)  [unwired: 2 in, 1 out]
          n154 = property on="HistoGraph" class="WFGraph (strict)"("Value"=w314, "Active Plot"=w316, "Plot.Plot Name"=w317) -> ()  [unwired: 2 in, 2 out]
        }
        n155 = property on="Binning" class="Ring (strict)"("StringsAndValues[]"=w289) -> ()  [unwired: 2 in, 2 out]
        n156 = local write "Channels"(w259) -> ()
        n157 = Bundle By Name(cluster=w285, "Channels"=w259, "SetInpChan"=w258, "SyncDivider"=w300, "SyncOffset"=w299, "SyncEdge"=w298, "SyncLevel"=w297, "UseDeadTime"=w263, "SyncDeadTime"=w262, "Binning"=w296, "HistoOffset"=w295, "AcqTime"=w294, "HistoLen"=w293, "StopOvl."=w292, "OvlLevel"=w291, "StartMeas"=w290, "Run cont."=w288) -> (w281:T4)
      }
      frame "SetInpChan" {
        n158 = Unbundle By Name(w326) -> ("DevIdx"=w321:i32, "Init Info.features"=w319:i32, "SetInpChan"=w324:T6[], "Channels"=w320:T3[])
        n159 = for {
          tunnel: w320 -> [w331]
          tunnel: w324 -> [w335] mode=indexing
          shift-right: [w333] -> w323
          shift-left: errorcluster {"status"=FALSE, "code"=0, "source"=""} ("error out") -> [w332]
          tunnel: w321 -> [w329]
          tunnel: w319 -> [w327]
          n160 = Unbundle By Name(w335) -> ("Cmds"=w334:T7[], "Channel"=w328:i32)
          n161 = Index Array(array=w331, index=w328) -> (element=w330:T3)
          n162 = for {
            tunnel: w334 -> [w342] mode=indexing
            tunnel: w328 -> [w341]
            shift-right: [w340] -> w333
            shift-left: w332 -> [w339]
            tunnel: w330 -> [w338]
            tunnel: w329 -> [w337]
            tunnel: w327 -> [w336]
            n163 = case shown="\"SetInpChanOffset\"" w342 {
              tunnel: w341 -> [_ w348 w355 w360 w376]
              tunnel: [w343 w347 w354 w364 w381] -> w340
              tunnel: w339 -> [w343 w346 w353 w363 w380]
              tunnel: w338 -> [_ w345 w352 w362 w379]
              tunnel: w337 -> [_ w344 w351 w361 w378]
              tunnel: w336 -> [_ _ _ w357 _]
              frame Default {
              }
              frame "SetInpChanEnable" {
                n164 = Unbundle By Name(w345) -> ("Enable"=w349:bool)
                n165 = call "MH_SetInputChannelEnable.vi"("error in (no error)"=w346, "enable"=w349, "channel"=w348, "devidx"=w344) -> ("error out"=w347:errorcluster)  [unwired: 6 in, 1 out]
              }
              frame "SetInpChanOffset" {
                n166 = Unbundle By Name(w352) -> ("Offset"=w350:i32)
                n167 = call "MH_SetInputChannelOffset.vi"("error in (no error)"=w353, "Offset"=w350, "channel"=w355, "devidx"=w351) -> ("error out"=w354:errorcluster)  [unwired: 6 in, 1 out]
              }
              frame "SetInpChanDeadTime" {
                w358 = 32  # FEATURE_PROG_TD
                n168 = And(x=w357, y=w358) -> (x .and. y?=w359:i32)
                n169 = Not Equal To 0?(x=w359) -> (x != 0?=w356:bool)
                n170 = case shown="False" w356 {
                  tunnel: [w365 w374] -> w364
                  tunnel: w363 -> [w365 w373]
                  tunnel: w362 -> [_ w372]
                  tunnel: w361 -> [_ w371]
                  tunnel: w360 -> [_ w369]
                  frame False {
                  }
                  frame True {
                    n171 = Unbundle By Name(w372) -> ("UseDeadTime"=w368:bool, "DeadTime"=w370:i32)
                    n172 = Boolean To (0,1)(Boolean=w368) -> (0, 1=w367:i16)
                    n173 = To Long Integer(number=w367) -> (32bit integer=w366:i32)
                    n174 = call "MH_SetInputDeadTime.vi"("channel"=w369, "error in (no error)"=w373, "deadtime"=w370, "on"=w366, "devidx"=w371) -> ("error out"=w374:errorcluster)  [unwired: 5 in, 1 out]
                  }
                }
              }
              frame "SetInpChanTrg" {
                n175 = Unbundle By Name(w379) -> ("Level"=w375:i32, "Edge"=w377:i32)
                n176 = call "MH_SetInputEdgeTrg.vi"("channel"=w376, "error in (no error)"=w380, "edge"=w377, "level"=w375, "devidx"=w378) -> ("error out"=w381:errorcluster)  [unwired: 5 in, 1 out]
              }
            }
          }
        }
      }
      frame "SetSyncDivider" {
        n177 = Unbundle By Name(w389) -> ("DevIdx"=w388:i32, "SyncDivider"=w384:i32)
        n178 = Power Of 2(x=w384) -> (2^x=w383:dbl)
        n179 = To Long Integer(number=w383) -> (32bit integer=w382:i32)
        n180 = call "MH_SetSyncDiv.vi"("SyncDivider"=w382, "devidx"=w388) -> ("error out"=w386:errorcluster)  [unwired: 8 in, 1 out]
        n181 = flat-sequence {
          tunnel: w386 -> [w390]
          tunnel: [w390] -> w385
          frame #0 {
            n182 = Wait (ms)(milliseconds to wait=u32 100) -> ()  [unwired: 1 out]
          }
        }
      }
      frame "SetSyncTrg" {
        n183 = Unbundle By Name(w397) -> ("DevIdx"=w394:i32, "SyncLevel"=w392:i32, "SyncEdge"=w393:i32)
        n184 = call "MH_SetSyncEdgeTrg.vi"("edge"=w393, "level"=w392, "devidx"=w394) -> ("error out"=w395:errorcluster)  [unwired: 7 in, 1 out]
      }
      frame "SetSyncDeadTime" {
        w400 = 32  # FEATURE_PROG_TD
        n185 = Unbundle By Name(w409) -> ("DevIdx"=w406:i32, "UseDeadTime"=w404:bool, "SyncDeadTime"=w405:i32, "Init Info.features"=w399:i32)
        n186 = Boolean To (0,1)(Boolean=w404) -> (0, 1=w403:i16)
        n187 = And(x=w399, y=w400) -> (x .and. y?=w401:i32)
        n188 = To Long Integer(number=w403) -> (32bit integer=w402:i32)
        n189 = Not Equal To 0?(x=w401) -> (x != 0?=w398:bool)
        n190 = case shown="False" w398 {
          tunnel: [_ w413] -> w407
          tunnel: w406 -> [_ w412]
          tunnel: w405 -> [_ w411]
          tunnel: w402 -> [_ w410]
          frame False {
          }
          frame True {
            n191 = call "MH_SetSyncDeadTime.vi"("deadtime"=w411, "on"=w410, "devidx"=w412) -> ("error out"=w413:errorcluster)  [unwired: 7 in, 1 out]
          }
        }
      }
      frame "SetSyncOffset" {
        n192 = Unbundle By Name(w418) -> ("DevIdx"=w416:i32, "SyncOffset"=w415:i32)
        n193 = call "MH_SetSyncChannelOffset.vi"("Offset"=w415, "devidx"=w416) -> ("error out"=w417:errorcluster)  [unwired: 8 in, 1 out]
      }
      frame "SetBinning" {
        # "When binning is changed the new resolution is querried"
        n194 = Unbundle By Name(w425) -> ("DevIdx"=w423:i32, "Binning"=w422:i32)
        n195 = call "MH_SetBinning.vi"("Binning"=w422, "devidx"=w423) -> ("error out"=w424:errorcluster)  [unwired: 8 in, 1 out]
        n196 = Build Array (concatenate)(MH_UIThread_Cmds."GetResolution", w420) -> (w421:T8[])
      }
      frame "SetHistoOffset" {
        n197 = Unbundle By Name(w430) -> ("DevIdx"=w427:i32, "HistoOffset"=w426:i32)
        n198 = call "MH_SetOffset.vi"("Offset"=w426, "devidx"=w427) -> ("error out"=w428:errorcluster)  [unwired: 8 in, 1 out]
      }
      frame "SetHistoLen" {
        n199 = Unbundle By Name(w433) -> ("DevIdx"=w435:i32, "HistoLen"=w434:i32)
        n200 = call "MH_SetHistoLen.vi"("lencode"=w434, "devidx"=w435) -> ("error out"=w436:errorcluster, "actuallen"=w431:i32)  [unwired: 7 in, 1 out]
        n201 = Bundle By Name(cluster=w433, "HistoLength"=w431) -> (w432:T4)
      }
      frame "SetStopOvl" {
        n202 = Unbundle By Name(w443) -> ("DevIdx"=w440:i32, "StopOvl."=w439:bool, "OvlLevel"=w438:u32)
        n203 = call "MH_SetStopOverflow.vi"("stopcount"=w438, "StopOnOverflow"=w439, "devidx"=w440) -> ("error out"=w441:errorcluster)  [unwired: 7 in, 1 out]
      }
      frame "GetAllRates" {
        # "An alternative to GetRates"
        n204 = Unbundle By Name(w452) -> ("DevIdx"=w449:i32, "Init Info.nchannels"=w444:i32)
        n205 = call "MH_AllocateCntRateBuffer.vi"("NumChan"=w444) -> ("Buffer"=w445:i32[])  [unwired: 10 in]
        n206 = call "MH_GetAllCountRates.vi"("cntrates_buf"=w445, "devidx"=w449) -> ("error out"=w446:errorcluster, "cntrates"=→"CountRates":i32[], "syncrate"=w448:i32)  [unwired: 6 in, 1 out]
        n207 = Format Into String(format string="Sync Rate: %d cps\n", w448) -> (resulting string=→"SyncRate":string)  [unwired: 2 in, 1 out]
      }
      frame "GetRates" {
        # "An alternative to GetAllRates"
        n208 = Unbundle By Name(w463) -> ("Init Info.nchannels"=w458:i32, "Channels"=w460:T3[], "DevIdx"=w459:i32)
        n209 = call "MH_GetSyncRate.vi"("devidx"=w459) -> ("error out"=w456:errorcluster, "syncrate"=w455:i32)  [unwired: 8 in, 1 out]
        n210 = Format Into String(format string="Sync Rate: %d cps\n", w455) -> (resulting string=w457:string)  [unwired: 2 in, 1 out]
        n211 = for {
          N: w458 -> [_]
          tunnel: w459 -> [w470]
          tunnel: [w467] -> w454 mode=indexing
          shift-right: [w469] -> w462
          shift-left: w456 -> [w471]
          tunnel: w460 -> [w466] mode=indexing
          i -> [w468]
          n212 = Unbundle By Name(w466) -> ("Enable"=w465:bool)
          n213 = case shown="True" w465 {
            tunnel: w471 -> [w472 w477]
            tunnel: w470 -> [_ w476]
            tunnel: [w472 w475] -> w469
            tunnel: w468 -> [_ w474]
            tunnel: [_ w473] -> w467
            frame False {
            }
            frame True {
              n214 = call "MH_GetCountRate.vi"("error in (no error)"=w477, "Channel"=w474, "devidx"=w476) -> ("error out"=w475:errorcluster, "rate"=w473:i32)  [unwired: 6 in, 1 out]
            }
          }
        }
        n215 = local write "SyncRate"(w457) -> ()
        n216 = local write "CountRates"(w454) -> ()
      }
      frame "StartMeas" {
        n217 = Unbundle By Name(w485) -> ("AcqTime"=w481:i32, "DevIdx"=w482:i32)
        n218 = call "MH_ClearHistMem.vi"("devidx"=w482) -> ("error out"=w483:errorcluster)  [unwired: 9 in, 1 out]
        n219 = call "MH_StartMeas.vi"("error in (no error)"=w483, "tacq"=w481, "devidx"=w482) -> ("error out"=w484:errorcluster)  [unwired: 7 in, 1 out]
        n220 = Build Array (concatenate)(w480, MH_UIThread_Cmds."GetAllHistos") -> (w479:T8[])
      }
      frame "StopMeas" {
        n221 = Unbundle By Name(w491) -> ("Run cont."=w486:bool, "DevIdx"=w492:i32)
        n222 = call "MH_StopMeas.vi"("devidx"=w492) -> ("error out"=w493:errorcluster)  [unwired: 9 in, 1 out]
        n223 = case shown="False" w486 {
          tunnel: w491 -> [w497 w499]
          tunnel: [w496 w499] -> w490
          tunnel: [w494 w498] -> w489
          frame False {
            w494 = T8[] [enum."GetAllHistos"] items=["Idle", "Init", "SetInpChan", "SetSyncDivider", "SetSyncTrg", "SetSyncOffset", "SetSyncDeadTime", "SetBinning", "SetHistoOffset", "SetHistoLen", "SetStopOvl", "SetBitShift", "SetHistoAcqTime", "GetRates", "GetAllRates", "StartMeas", "StopMeas", "AbortMeas", "GetResolution", "GetHistos", "GetAllHistos", "ReadFiFo", "WriteStatus", "Resize", "EnableControls", "DisableControls", "Error", "Exit"]
            w495 = FALSE ("StartMeas")
            n224 = Bundle By Name(cluster=w497, "StartMeas"=w495) -> (w496:T4)
            n225 = local write "Start"(w495) -> ()
          }
          frame True {
            w498 = T8[] [enum."GetAllHistos", enum."StartMeas"] items=["Idle", "Init", "SetInpChan", "SetSyncDivider", "SetSyncTrg", "SetSyncOffset", "SetSyncDeadTime", "SetBinning", "SetHistoOffset", "SetHistoLen", "SetStopOvl", "SetBitShift", "SetHistoAcqTime", "GetRates", "GetAllRates", "StartMeas", "StopMeas", "AbortMeas", "GetResolution", "GetHistos", "GetAllHistos", "ReadFiFo", "WriteStatus", "Resize", "EnableControls", "DisableControls", "Error", "Exit"]
          }
        }
        n226 = Build Array (concatenate)(w488, w489) -> (w487:T8[])
      }
      frame "AbortMeas" {
        w503 = T8[] [enum."GetAllHistos"] items=["Idle", "Init", "SetInpChan", "SetSyncDivider", "SetSyncTrg", "SetSyncOffset", "SetSyncDeadTime", "SetBinning", "SetHistoOffset", "SetHistoLen", "SetStopOvl", "SetBitShift", "SetHistoAcqTime", "GetRates", "GetAllRates", "StartMeas", "StopMeas", "AbortMeas", "GetResolution", "GetHistos", "GetAllHistos", "ReadFiFo", "WriteStatus", "Resize", "EnableControls", "DisableControls", "Error", "Exit"]
        w500 = FALSE ("StartMeas")
        n227 = Unbundle By Name(w505) -> ("DevIdx"=w506:i32)
        n228 = call "MH_StopMeas.vi"("devidx"=w506) -> ("error out"=w507:errorcluster)  [unwired: 9 in, 1 out]
        n229 = Bundle By Name(cluster=w505, "StartMeas"=w500) -> (w504:T4)
        n230 = local write "Start"(w500) -> ()
        n231 = Build Array (concatenate)(w502, w503) -> (w501:T8[])
      }
      frame "GetResolution" {
        # "Resolution in ns"
        # "Gets resolution in ps"
        # "Resolution is saved in UIThread Data cluster in ns"
        n232 = Unbundle By Name(w512) -> ("DevIdx"=w514:i32)
        n233 = call "MH_GetResolution.vi"("devidx"=w514) -> ("error out"=w513:errorcluster, "resolution"=w510:dbl)  [unwired: 8 in, 1 out]
        n234 = Divide(x=w510, y=1000.0) -> (x/y=w508:dbl)
        n235 = Bundle By Name(cluster=w512, "Resolution"=w508) -> (w511:T4)
      }
      frame "GetAllHistos" {
        w528 = 1  # FLAG_OVERFLOW
        # "Provides a buffer (U32-array of length 'HistoLength' x nchannels) for all histograms."
        # "An alternative to GetHistos"
        n236 = Unbundle By Name(w539) -> ("Resolution"=w538:dbl, "DevIdx"=w518:i32, "HistoLength"=w521:i32, "Init Info.nchannels"=w522:i32)
        n237 = call "MH_AllocateAllHistoBuffer.vi"("NumChan"=w522, "HistoLength"=w521) -> ("Buffer"=w519:u32[])  [unwired: 9 in]
        n238 = call "MH_GetAllHistograms.vi"("Chcount"=w519, "devidx"=w518) -> ("error out"=w516:errorcluster, "Histograms"=w517:u32[])  [unwired: 7 in, 1 out]
        n239 = Reshape Array(w517, w522, w521) -> (w520:u32[][])
        n240 = for {
          tunnel: [w541] -> w530 mode=indexing
          shift-right: [w543] -> w524
          shift-left: "Total Counts:\t\t" -> [w542]
          tunnel: w520 -> [w541] mode=indexing
          i -> [w547]
          n241 = Add Array Elements(numeric array=w541) -> (sum=w544:u32)
          n242 = Increment(x=w547) -> (x+1=w545:i32)
          n243 = Format Into String(format string="Ch.%2d: %d cnts.\t\t", initial string=w542, w545, w544) -> (resulting string=w543:string)  [unwired: 1 in, 1 out]
        }
        n244 = call "CalcRate.vi"("Refresh(ms)"=u32 500) -> ("Rate / Hz"=w536:dbl)  [unwired: 8 in, 2 out]
        n245 = Format Into String(format string="Readout Rate: %.1f Hz\\t\\t", w536) -> (resulting string=w534:string)  [unwired: 2 in, 1 out]
        n246 = Concatenate Strings(w534, w524) -> (w533:string)
        n247 = Bundle(0.0, "Resolution"=w538, "Histograms"=w530) -> (→"HistoGraph":T13)  [unwired: 1 in]
        n248 = local write "Status"(w533) -> ()
        n249 = call "MH_GetFlags.vi"("error in (no error)"=w516) -> ("error out"=w537:errorcluster, "flags"=w527:i32)  [unwired: 8 in, 1 out]
        n250 = And(x=w528, y=w527) -> (x .and. y?=w529:i32)
        n251 = Not Equal To 0?(x=w529) -> (x != 0?=→"OverFlow":bool)
      }
      frame "GetHistos" {
        w557 = 1  # FLAG_OVERFLOW
        # "Provides a buffer (U32-array of length 'HistoLength') for histograms."
        # "An alternative to GetAllHistos"
        n252 = Unbundle By Name(w571) -> ("Resolution"=w568:dbl, "Init Info.nchannels"=w550:i32, "Channels"=w551:T3[], "DevIdx"=w570:i32, "HistoLength"=w569:i32)
        n253 = call "MH_AllocateHistoBuffer.vi"("HistoLength"=w569) -> ("Buffer"=w562:u32[])  [unwired: 10 in]
        n254 = for {
          N: w550 -> [_]
          tunnel: w570 -> [w585]
          tunnel: [w573] -> w560 mode=indexing
          tunnel: w562 -> [w583]
          shift-right: [w584] -> w559
          shift-left: errorcluster {"status"=FALSE, "code"=0, "source"=""} ("error IO") -> [w577]
          shift-right: [w578] -> w553
          shift-left: "Total Counts:\t\t" -> [w576]
          tunnel: w551 -> [w575] mode=indexing
          i -> [w582]
          n255 = Unbundle By Name(w575) -> ("Enable"=w574:bool)
          n256 = case shown="True" w574 {
            tunnel: w585 -> [_ w593]
            tunnel: [w586 w592] -> w584
            tunnel: w583 -> [w587 w591]
            tunnel: [w587 w590] -> w573
            tunnel: w582 -> [_ w589]
            tunnel: w577 -> [w586 w588]
            frame False {
            }
            frame True {
              n257 = call "MH_GetHistogram.vi"("Chcount"=w591, "error in (no error)"=w588, "channel"=w589, "devidx"=w593) -> ("error out"=w592:errorcluster, "Histogram"=w590:u32[])  [unwired: 5 in, 1 out]
            }
          }
          n258 = Add Array Elements(numeric array=w573) -> (sum=w579:u32)
          n259 = Increment(x=w582) -> (x+1=w580:i32)
          n260 = Format Into String(format string="Ch.%2d: %d cnts.\t\t", initial string=w576, w580, w579) -> (resulting string=w578:string)  [unwired: 1 in, 1 out]
        }
        n261 = call "CalcRate.vi"("Refresh(ms)"=u32 500) -> ("Rate / Hz"=w566:dbl)  [unwired: 8 in, 2 out]
        n262 = Format Into String(format string="Readout Rate: %.1f Hz\\t\\t", w566) -> (resulting string=w564:string)  [unwired: 2 in, 1 out]
        n263 = Concatenate Strings(w564, w553) -> (w563:string)
        n264 = Bundle(0.0, "Resolution"=w568, "Histogram"=w560) -> (w548:T2)  [unwired: 1 in]
        n265 = local write "HistoGraph"(w548) -> ()
        n266 = local write "Status"(w563) -> ()
        n267 = call "MH_GetFlags.vi"("error in (no error)"=w559) -> ("error out"=w567:errorcluster, "flags"=w556:i32)  [unwired: 8 in, 1 out]
        n268 = And(x=w557, y=w556) -> (x .and. y?=w558:i32)
        n269 = Not Equal To 0?(x=w558) -> (x != 0?=w549:bool)
        n270 = local write "OverFlow"(w549) -> ()
      }
      frame "WriteStatus" {
        n271 = Unbundle By Name(w595) -> ("Status"=→"Status":string)
      }
      frame "Resize" {
        n272 = property on="Pane 3" class="Pane"() -> ("Width"=w602:u32)  [unwired: 2 in, 2 out]
        n273 = Subtract(x=w602, y=i16 100 ("b")) -> (x-y=w608:u32)
        n274 = Unbundle By Name(w597) -> ("Init Info.nchannels"=w605:i32)
        n275 = Quotient & Remainder(x=w608, y=i16 99 ("m")) -> (floor(x/y)=w607:u32)  [unwired: 1 out]
        n276 = In Range and Coerce(upper limit=w605, x=w607, lower limit=4) -> (coerced(x)=w606:u32)  [unwired: 1 out]
        n277 = Equal?(x=w605, y=w606) -> (x = y?=w604:bool)
        n278 = Not(x=w604) -> (.not. x?=w603:bool)
        n279 = property on="Channels" class="Arr (strict)"("HorizScroll"=w603, "Number of Columns"=w606, "Index Values"=u32[] [0]) -> ()  [unwired: 2 in, 2 out]
      }
      frame "EnableControls" {
        n280 = property class="VI"() -> ("Panel"=w613:refnum<vi>)  [unwired: 2 in, 2 out]
        n281 = property class="Pnl"(reference=w613) -> ("Controls[]"=w612:refnum<vi>[])  [unwired: 1 in, 2 out]
        n282 = property class="Pnl"(reference=w613) -> ("Decos[]"=w614:refnum<vi>[])  [unwired: 1 in, 2 out]
        n283 = for {
          tunnel: w614 -> [w618] mode=indexing
          tunnel: TRUE -> [w617]
          n284 = property class="Decor"(reference=w618, "Visible"=w617) -> ()  [unwired: 1 in, 2 out]
        }
        n285 = for {
          tunnel: w612 -> [w621] mode=indexing
          tunnel: T9."Enabled" ("Disabled") -> [w620]
          tunnel: [w619] -> _
          n286 = property class="Ctl"(reference=w621, "DisabledEnum"=w620) -> (error out=w619:errorcluster)  [unwired: 1 in, 1 out]
        }
      }
      frame "DisableControls" {
        n287 = property class="VI"() -> ("Panel"=w625:refnum<vi>)  [unwired: 2 in, 2 out]
        n288 = property class="Pnl"(reference=w625) -> ("Controls[]"=w624:refnum<vi>[])  [unwired: 1 in, 2 out]
        n289 = property class="Pnl"(reference=w625) -> ("Decos[]"=w626:refnum<vi>[])  [unwired: 1 in, 2 out]
        n290 = for {
          tunnel: w626 -> [w630] mode=indexing
          tunnel: FALSE -> [w629]
          n291 = property class="Decor"(reference=w630, "Visible"=w629) -> ()  [unwired: 1 in, 2 out]
        }
        n292 = for {
          tunnel: w624 -> [w633] mode=indexing
          tunnel: T9."Disabled and Grayed Out" ("Disabled") -> [w632]
          tunnel: [w631] -> _
          n293 = property class="Ctl"(reference=w633, "DisabledEnum"=w632) -> (error out=w631:errorcluster)  [unwired: 1 in, 1 out]
        }
      }
      frame "Error" {
        w634 = T8[] [enum."Exit"] items=["Idle", "Init", "SetInpChan", "SetSyncDivider", "SetSyncTrg", "SetSyncOffset", "SetSyncDeadTime", "SetBinning", "SetHistoOffset", "SetHistoLen", "SetStopOvl", "SetBitShift", "SetHistoAcqTime", "GetRates", "GetAllRates", "StartMeas", "StopMeas", "AbortMeas", "GetResolution", "GetHistos", "GetAllHistos", "ReadFiFo", "WriteStatus", "Resize", "EnableControls", "DisableControls", "Error", "Exit"]
        w637 = T14 1 items=["no dialog", "OK message", "continue or stop message", "OK message + warnings", "continue/stop + warnings"] ("type of dialog (OK msg:1)")
        # "Error case: If an error occures the user is informed and the programm terminates. Add your own code to handle error events (e.g. exception lists, etc.)"
        n294 = call <vilib>:"Simple Error Handler.vi"("type of dialog (OK msg:1)"=w637, "error in (no error)"=w636) -> ()  [unwired: 3 in, 5 out]
      }
      frame "Exit" {
        n295 = Unbundle By Name(w641) -> ("DevIdx"=w640:i32)
        n296 = call "MH_CloseDevice.vi"("devidx"=w640) -> ("error out"=w639:errorcluster)  [unwired: 9 in, 1 out]
      }
    }
    n297 = call "MH_EnQError.vi"("error in (no error)"=w8, "Cmds_in"=w6) -> ("error out"=w7:errorcluster, "Cmds_out"=w5:T8[])  [unwired: 8 in]
  }
